vi "Parse SYS_STATUS.vi"(11 "Data":string) -> (3 "System Status":T1)   [LabVIEW 2014]
uses:
  Controls/MAVLink System Status.ctl
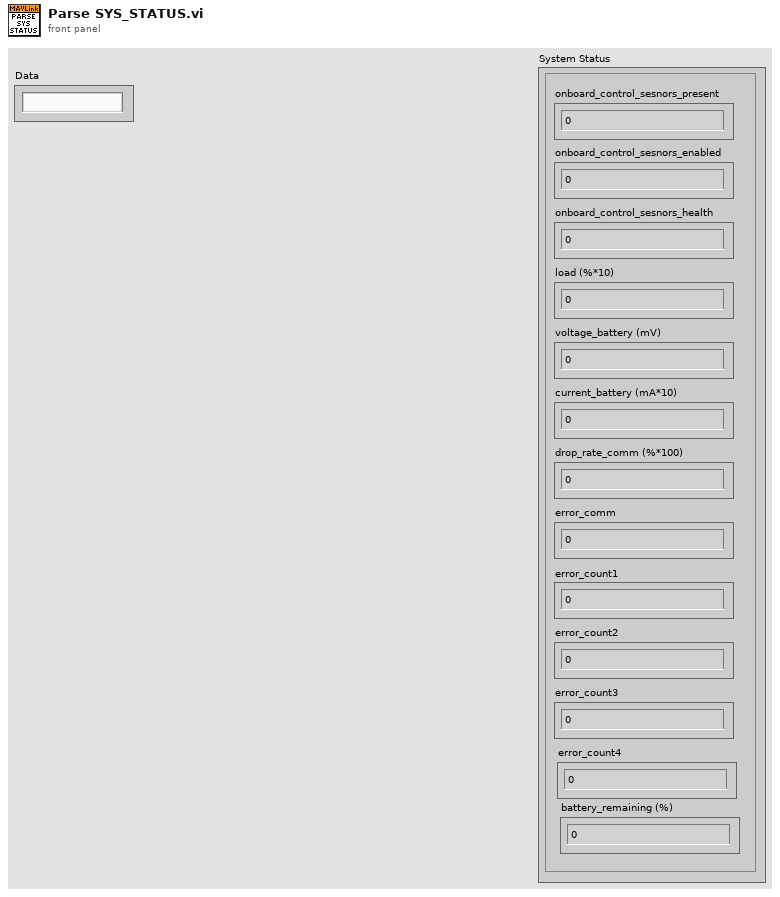
[diagram p1: front panel]
types:
  T1 = typedef "MAVLink System Status.ctl" = cluster{"onboard_control_sesnors_present":u32, "onboard_control_sesnors_enabled":u32, "onboard_control_sesnors_health":u32, "load (%*10)":u16, "voltage_battery (mV)":u16, "current_battery (mA*10)":i16, "drop_rate_comm (%*100)":u16, "error_comm":u16, "error_count1":u16, "error_count2":u16, "error_count3":u16, "error_count4":u16, "battery_remaining (%)":i8}
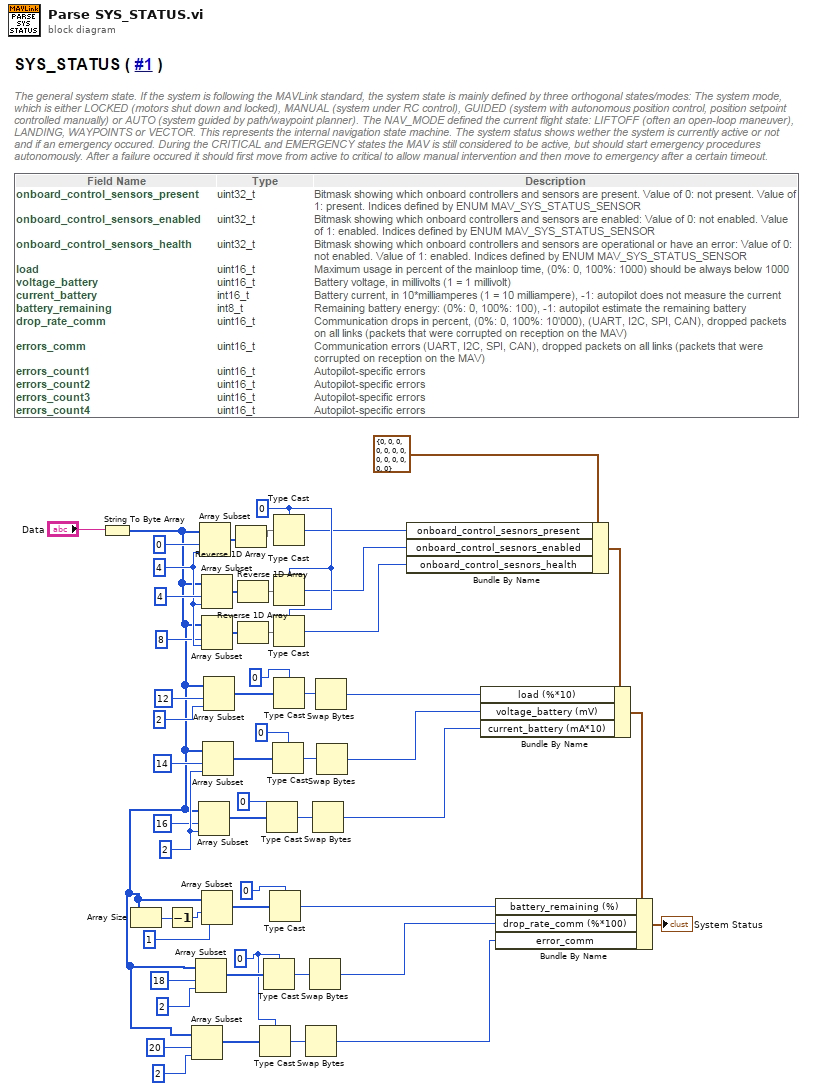
[diagram p0: block diagram]
diagram:
  w9 = u16 0
  w33 = 2 ("length")
  w43 = u32 0
  w46 = 4 ("length")
  n1 = String To Byte Array(string="Data") -> (unsigned byte array=w6:u8[])
  n2 = Array Size(array=w6) -> (size(s)=w18:i32)
  n3 = Decrement(x=w18) -> (x-1=w17:i32)
  n4 = Array Subset(array=w6, index=20, length=2) -> (w8:u8[])
  n5 = Array Subset(array=w6, index=18, length=2) -> (w13:u8[])
  n6 = Array Subset(array=w6, index=16, length=w33) -> (w37:u8[])
  n7 = Array Subset(array=w6, index=0, length=w46) -> (w53:u8[])
  n8 = Array Subset(array=w6, index=4, length=w46) -> (w47:u8[])
  n9 = Array Subset(array=w6, index=8, length=w46) -> (w48:u8[])
  n10 = Array Subset(array=w6, index=w17, length=1) -> (w20:u8[])
  n11 = Array Subset(array=w6, index=14, length=w33) -> (w34:u8[])
  n12 = Array Subset(array=w6, index=12, length=2) -> (w30:u8[])
  n13 = Reverse 1D Array(array=w53) -> (reversed array=w54:u8[])
  n14 = Reverse 1D Array(array=w47) -> (reversed array=w52:u8[])
  n15 = Reverse 1D Array(array=w48) -> (reversed array=w49:u8[])
  n16 = Type Cast(type=w9, x=w8) -> (*(type *) &x=w7:u16)
  n17 = Type Cast(type=w9, x=w13) -> (*(type *) &x=w14:u16)
  n18 = Type Cast(type=i16 0, x=w37) -> (*(type *) &x=w38:i16)
  n19 = Type Cast(type=i8 0, x=w20) -> (*(type *) &x=w4:i8)
  n20 = Type Cast(type=u16 0, x=w34) -> (*(type *) &x=w26:u16)
  n21 = Type Cast(type=w43, x=w54) -> (*(type *) &x=w42:u32)
  n22 = Type Cast(type=w43, x=w52) -> (*(type *) &x=w41:u32)
  n23 = Type Cast(type=w43, x=w49) -> (*(type *) &x=w40:u32)
  n24 = Type Cast(type=u16 0, x=w30) -> (*(type *) &x=w27:u16)
  n25 = Swap Bytes(anything=w7) -> (byte swapped=w2:u16)
  n26 = Swap Bytes(anything=w14) -> (byte swapped=w3:u16)
  n27 = Swap Bytes(anything=w38) -> (byte swapped=w22:i16)
  n28 = Swap Bytes(anything=w27) -> (byte swapped=w24:u16)
  n29 = Swap Bytes(anything=w26) -> (byte swapped=w23:u16)
  n30 = Bundle By Name(cluster=T1 {"onboard_control_sesnors_present"=0, "onboard_control_sesnors_enabled"=0, "onboard_control_sesnors_health"=0, "load (%*10)"=0, "voltage_battery (mV)"=0, "current_battery (mA*10)"=0, "drop_rate_comm (%*100)"=0, "error_comm"=0, "error_count1"=0, "error_count2"=0, "error_count3"=0, "error_count4"=0, "battery_remaining (%)"=0} ("System Status"), "onboard_control_sesnors_present"=w42, "onboard_control_sesnors_enabled"=w41, "onboard_control_sesnors_health"=w40) -> (w21:T1)
  n31 = Bundle By Name(cluster=w21, "load (%*10)"=w24, "voltage_battery (mV)"=w23, "current_battery (mA*10)"=w22) -> (w5:T1)
  n32 = Bundle By Name(cluster=w5, "battery_remaining (%)"=w4, "drop_rate_comm (%*100)"=w3, "error_comm"=w2) -> (→"System Status":T1)
